vi "Get Name.vi"(8 "error in (no error)":errorcluster, 11 "Dependency Source_Custom in":refnum<class "Dependency Source_NIPM.lvclass">) -> (0 "error out":errorcluster, 2 "Dependency Source Name":string, 3 "Dependency Source_Custom out":refnum<class "Dependency Source_NIPM.lvclass">)   [LabVIEW 2019, in "Project.Dependencies Finder.lvlib" / "Dependency Source_NIPM.lvclass"]
doc: "Return the name of the dependency source. \n\nThis implementation returns 'NIPM'."
uses:
  Dependency Source_NIPM.lvclass
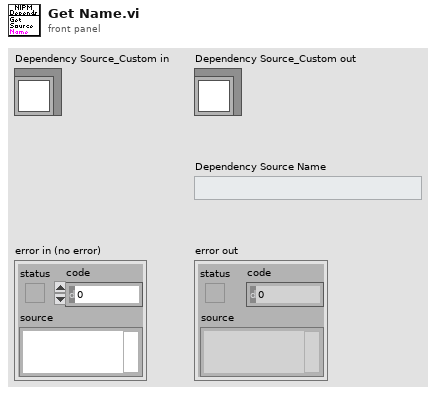
[diagram p1: front panel]
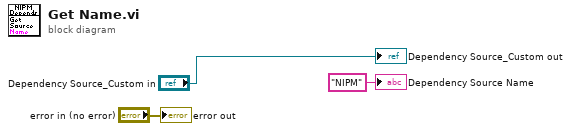
[diagram p0: block diagram]
diagram:
  "error out" <- "error in (no error)"
  "Dependency Source Name" <- "NIPM" ("Dependency Source Name")
  "Dependency Source_Custom out" <- "Dependency Source_Custom in"
